vi "运维调试_采配水V1.vi"() -> ()   [LabVIEW 2016, in "PLC.lvlib"]
uses:
  PLC.lvlib
  <vilib>/Plasmionique/MB Master/MB_Master/MB_Master.lvclass
  <vilib>/Utility/miscctls.llb/LVPointTypeDef.ctl
  <vilib>/Plasmionique/MB Master/MB_Master_Serial/MB_Master_Serial.lvclass
  C:/Program Files (x86)/National Instruments/LabVIEW 2016/vi.lib/Plasmionique/MB Master/MB_Master/MB_Master.lvclass
  <vilib>/Instr/_visa.llb/VISA Configure Serial Port (Instr).vi
  <vilib>/NI/Modbus Library/API/Wrapper/Create TCP Slave.vi
  <vilib>/NI/Modbus Library/API/Slave/Modbus Slave.lvclass
  <vilib>/Plasmionique/MB Master/MB Master.lvlib
  <vilib>/NI/Modbus Library/API/Wrapper/API Main.lvlib
panel:
  out "Registers":u16[](array[numeric])
  out "R118":i16 caption="多参数沉淀时间"
  in  "下载模式":bool
  out "当前启动泵号":u16(ring) items=["1号水样泵", "2号水样泵"]
  out "R113":i16 caption="储水时间设定"
  out "X2":bool caption="X1"
  out "采配水版本号":string
  out "R23":i16 caption="清洗频次计数"
  out "R112":i16 caption="清洗频次设定"
  out "R22":i16
  in  "Y15":bool
  out "R111":i16 caption="排液时间"
  out "通讯故障":bool
  out "R21":i16
  in  "Y14":bool
  out "R20":i16
  in  "Y13":bool
  in  "潜水泵工作模式":u16(ring) items=["泵1单泵单管路", "泵2单泵单管路", "潜水泵双泵双管路", "自吸泵双泵双管路"]
  out "X10":bool caption="废液报警"
  out "X9":bool caption="自来水检测"
  out "X8":bool caption="泵2过载报警"
  out "X7":bool caption="泵1过载报警"
  out "X6":bool caption="断电检测"
  out "X5":bool caption="开门检测"
  out "X4":bool caption="烟雾检测"
  out "X3":bool caption="漏水检测"
  out "X1":bool
  out "X0":bool caption="采样池液位开关"
  out "R109":i16 caption="配水时间"
  out "集成报警信息":string
  out "R108":i16 caption="自来水报警"
  out "R107":i16 caption="采水池液位报警设置"
  out "R106":i16 caption="进样超时设置"
  out "R105":i16 caption="二级清洗时间"
  out "R104":i16 caption="一级清洗时间"
  out "R103":i16 caption="外部管路清洗时间"
  out "R102":i16 caption="静置沉淀时间"
  out "R101":i16 caption="内部管路润洗时间"
  out "R100":i16 caption="外部管路润洗时间"
  out "R2":i16
  out "R1":i16
  out "多列列表框":i32(listbox)
  out "R19":i16
  in  "Y7":bool
  out "R18":i16
  in  "Y6":bool
  out "R17":i16
  in  "Y5":bool
  out "R16":i16
  in  "Y4":bool
  out "R15":i16
  in  "Y3":bool
  out "R14":i16
  in  "Y2":bool
  out "R13":i16
  in  "Y1":bool
  out "R12":i16
  in  "Y0":bool
  in  "返回":bool
  in  "参数设置":bool
  in  "单步启动":bool
  in  "启动":bool
  in  "停止":bool
  # "S"
  # "S"
  # "次"
  # "次"
  # "S"
  # "S"
  # "S"
  # "S"
  # "S"
  # "S"
  # "S"
  # "S"
  # "S"
  # "S"
  # "S"
  # "单步计时："
  # "s"
  # "流程计时："
  # "s"
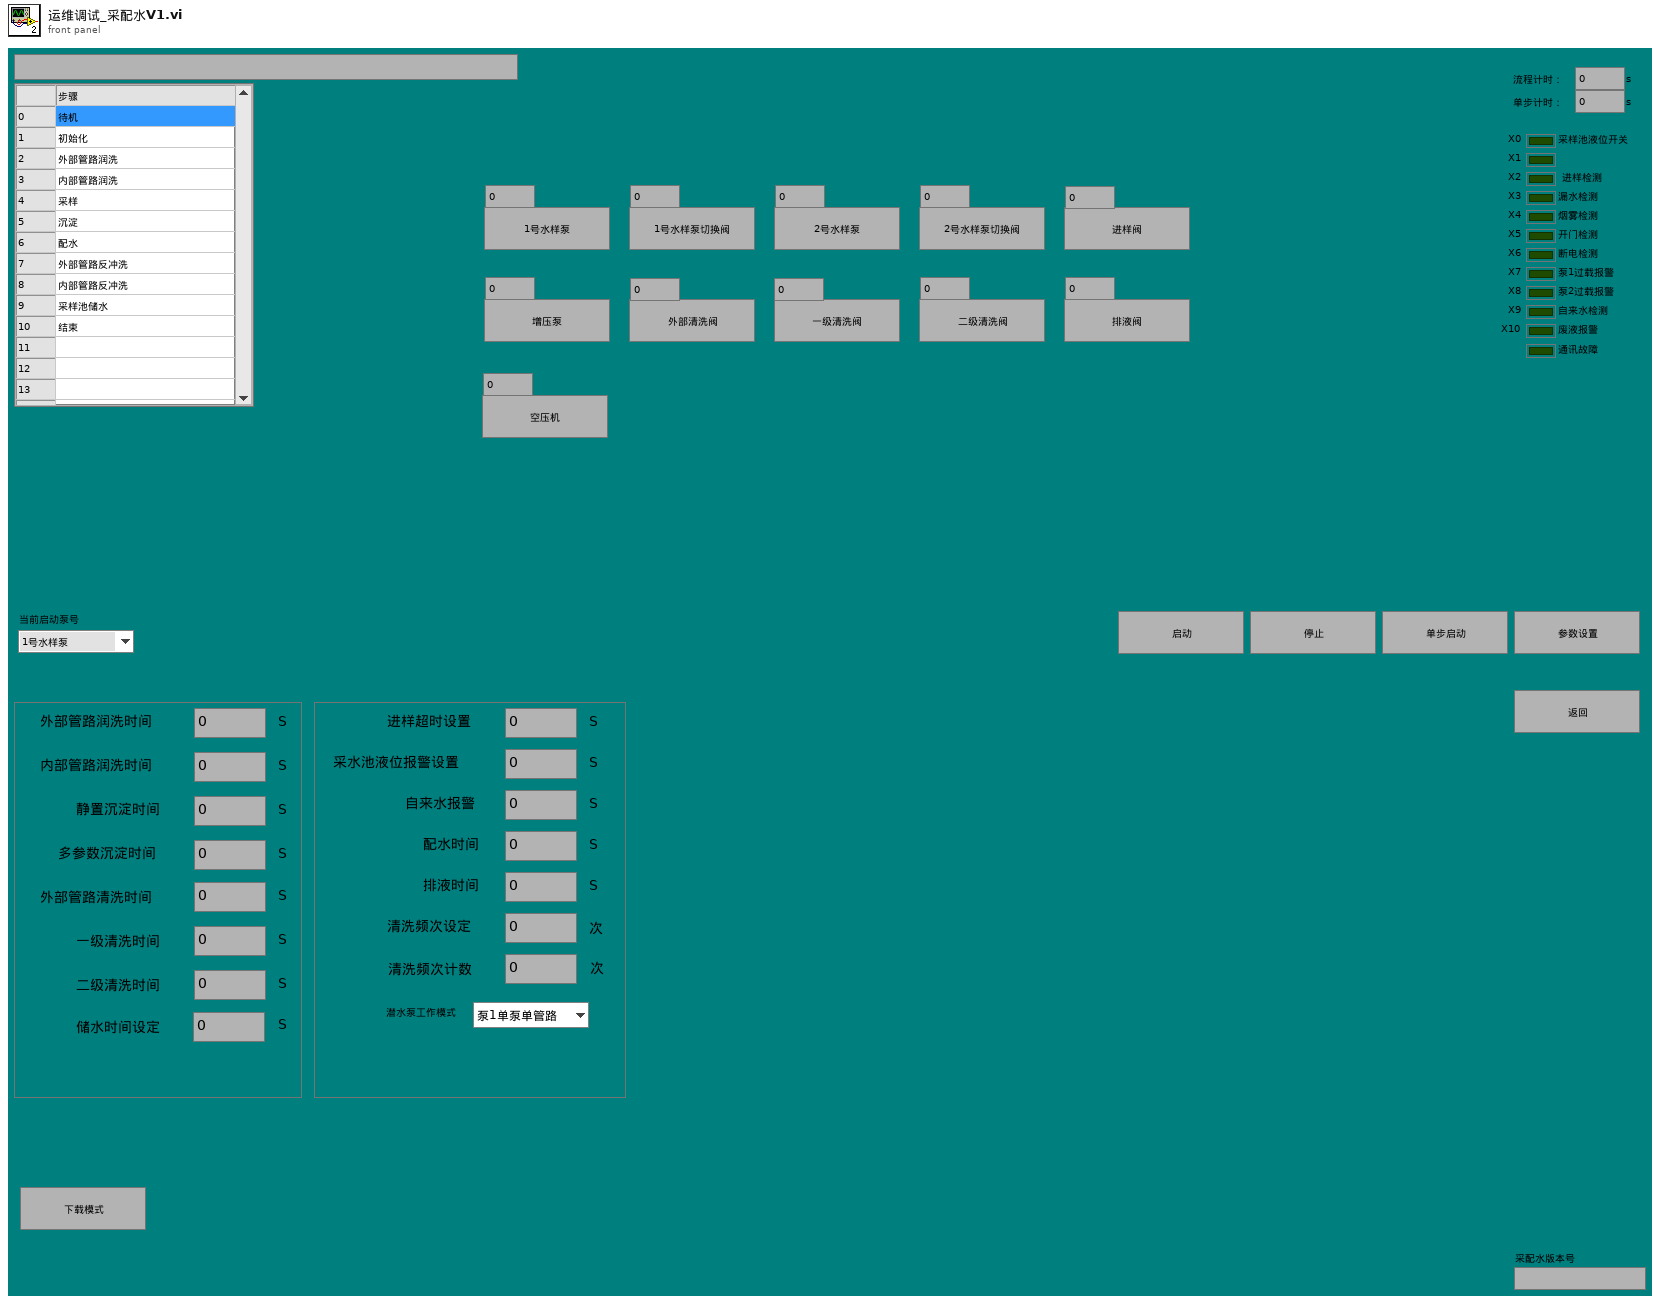
[diagram p1: front panel]
types:
  T1 = typedef "LVPointTypeDef.ctl" = cluster{"Horizontal":i16, "Vertical":i16}
  T2 = cluster{"命令":string, "数据":cluster{"starting address":u16, "holding register value":u16}}
  T3 = cluster{"时间标识":timestamp, "设备":string, "日志信息":string}
  T4 = cluster{"R0":i16, "R1":i16, "R2":i16, "R3":i16, "R4":i16, "R5":i16, "R6":i16, "R7":i16, "R8":i16, "R9":i16, "R10":i16, "R11":i16, "R12":i16, "R13":i16, "R14":i16, "R15":i16, "R16":i16, "R17":i16, "R18":i16, "R19":i16, "R20":i16, "R21":i16, "R22":i16, "R23":i16, "R24":i16, "R25":i16, "R26":i16, "R27":i16, "R28":i16, "R29":i16, "R30":i16, "R31":i16, "R32":i16, "R33":i16, "R34":i16}
  T5 = cluster{"seconds since 1Jan1904":timestamp, "table输入":string, string, "table输入":string}
  T6 = cluster{"时间标识":timestamp, "设备":string, "日志信息":string, "流程参数":string}
  T7 = cluster{"命令":string, cluster{"starting address":u16, "holding register value":u16}}
  T8 = cluster{"命令":string, "数据":cluster{"starting address":u16, "holding register values":u16[]}}
  T9 = cluster{"命令":string, "data":cluster{"starting address":u16, "coil values":bool[]}}
  T10 = cluster{"测试模式":enum16{"正常测试", "集成干预"}, "参数启用":cluster{"氨氮":bool, "总磷总氮":bool, "CODMn":bool, "CODcr":bool, "多参数":bool, "超标留样":bool}}
  T11 = enum32{"Bad", "Idle", "Run top level", "Running"}
  T12 = cluster{"baud rate (bps)":u32, "stop bits":u16, "parity":u16, "flow control":u16, "timeout":u32, "retries":i32}
  T13 = cluster{"starting address":u16, "holding register values":u16[]}
  T14 = cluster{"starting address":u16, "holding register value":u16}
  T15 = cluster{"starting address":u16, "coil values":bool[]}
  T16 = cluster{"Registers[0]":u16, "Registers[1]":u16, "Registers[2]":u16, "Registers[3]":u16, "Registers[4]":u16, "Registers[5]":u16, "Registers[6]":u16, "Registers[7]":u16, "Registers[8]":u16, "Registers[9]":u16, "Registers[10]":u16, "Registers[11]":u16, "Registers[12]":u16, "Registers[13]":u16, "Registers[14]":u16, "Registers[15]":u16, "Registers[16]":u16, "Registers[17]":u16, "Registers[18]":u16, "Registers[19]":u16, "Registers[20]":u16, "Registers[21]":u16, "Registers[22]":u16, "Registers[23]":u16, "Registers[24]":u16, "Registers[25]":u16, "Registers[26]":u16, "Registers[27]":u16, "Registers[28]":u16, "Registers[29]":u16, "Registers[30]":u16, "Registers[31]":u16, "Registers[32]":u16, "Registers[33]":u16, "Registers[34]":u16}
  T17 = cluster{"Registers[0]":u16, "Registers[1]":u16, "Registers[2]":u16, "Registers[3]":u16, "Registers[4]":u16, "Registers[5]":u16}
  T18 = cluster{"Registers[0]":u16, "Registers[1]":u16, "Registers[2]":u16, "Registers[3]":u16, "Registers[4]":u16, "Registers[5]":u16, "Registers[6]":u16, "Registers[7]":u16, "Registers[8]":u16, "Registers[9]":u16, "Registers[10]":u16, "Registers[11]":u16, "Registers[12]":u16, "Registers[13]":u16, "Registers[14]":u16, "Registers[15]":u16, "Registers[16]":u16, "Registers[17]":u16, "Registers[18]":u16, "Registers[19]":u16}
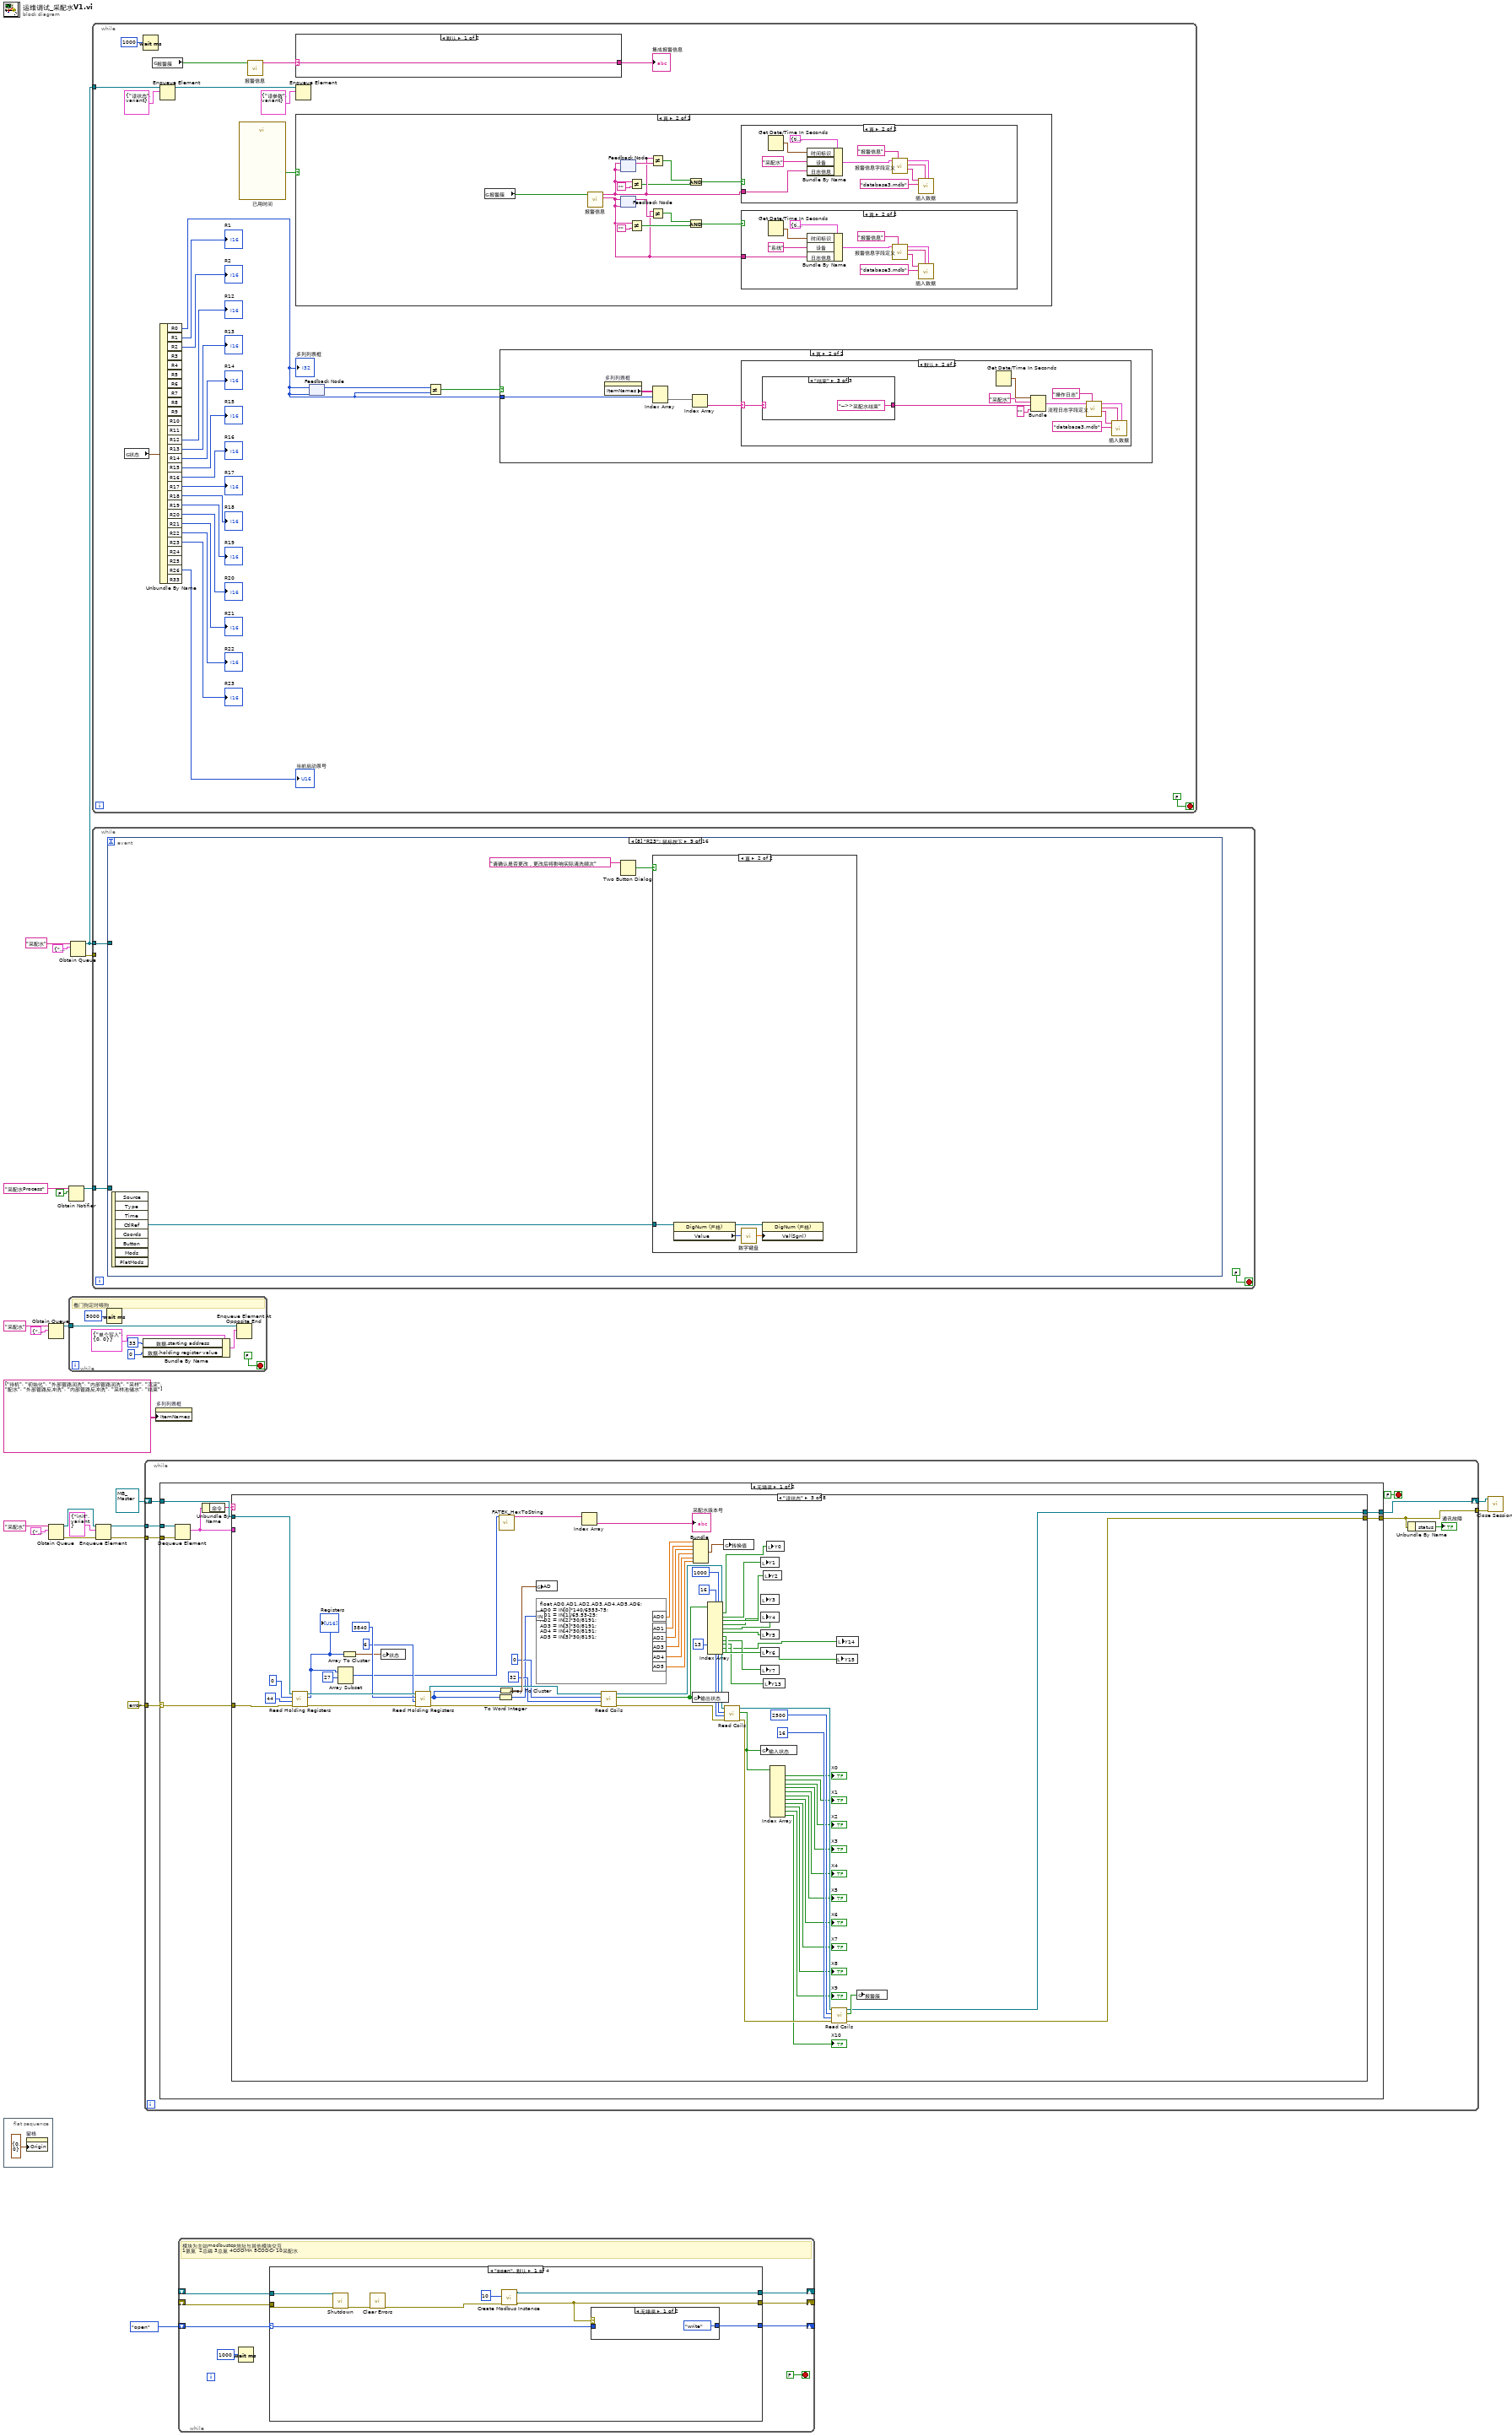
[diagram p0: block diagram]
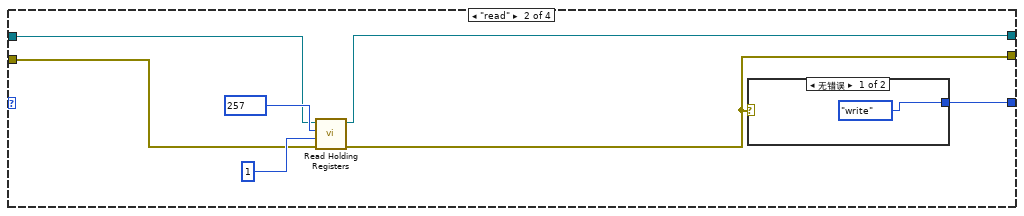
[diagram p3: hidden frame]
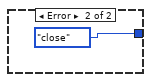
[diagram p4: hidden frame]
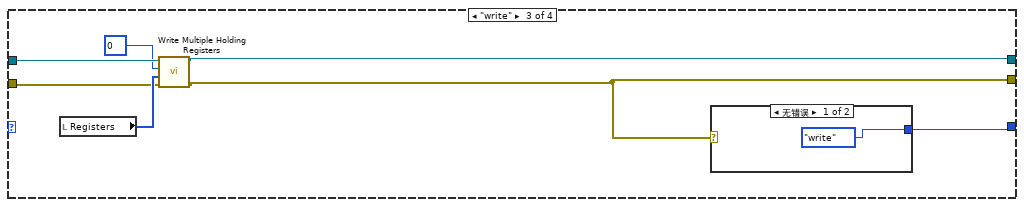
[diagram p5: hidden frame]
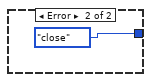
[diagram p6: hidden frame]
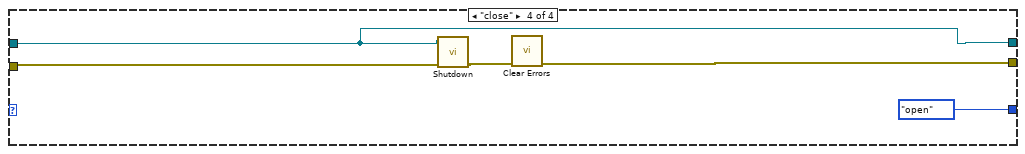
[diagram p7: hidden frame]
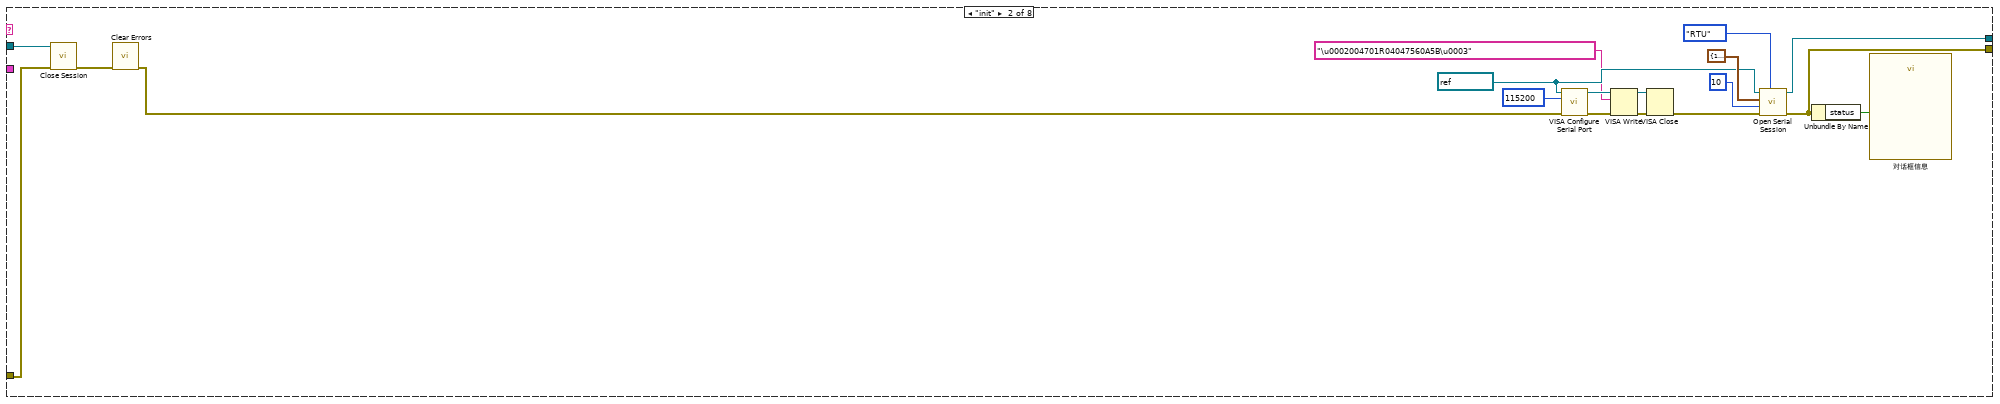
[diagram p9: hidden frame]
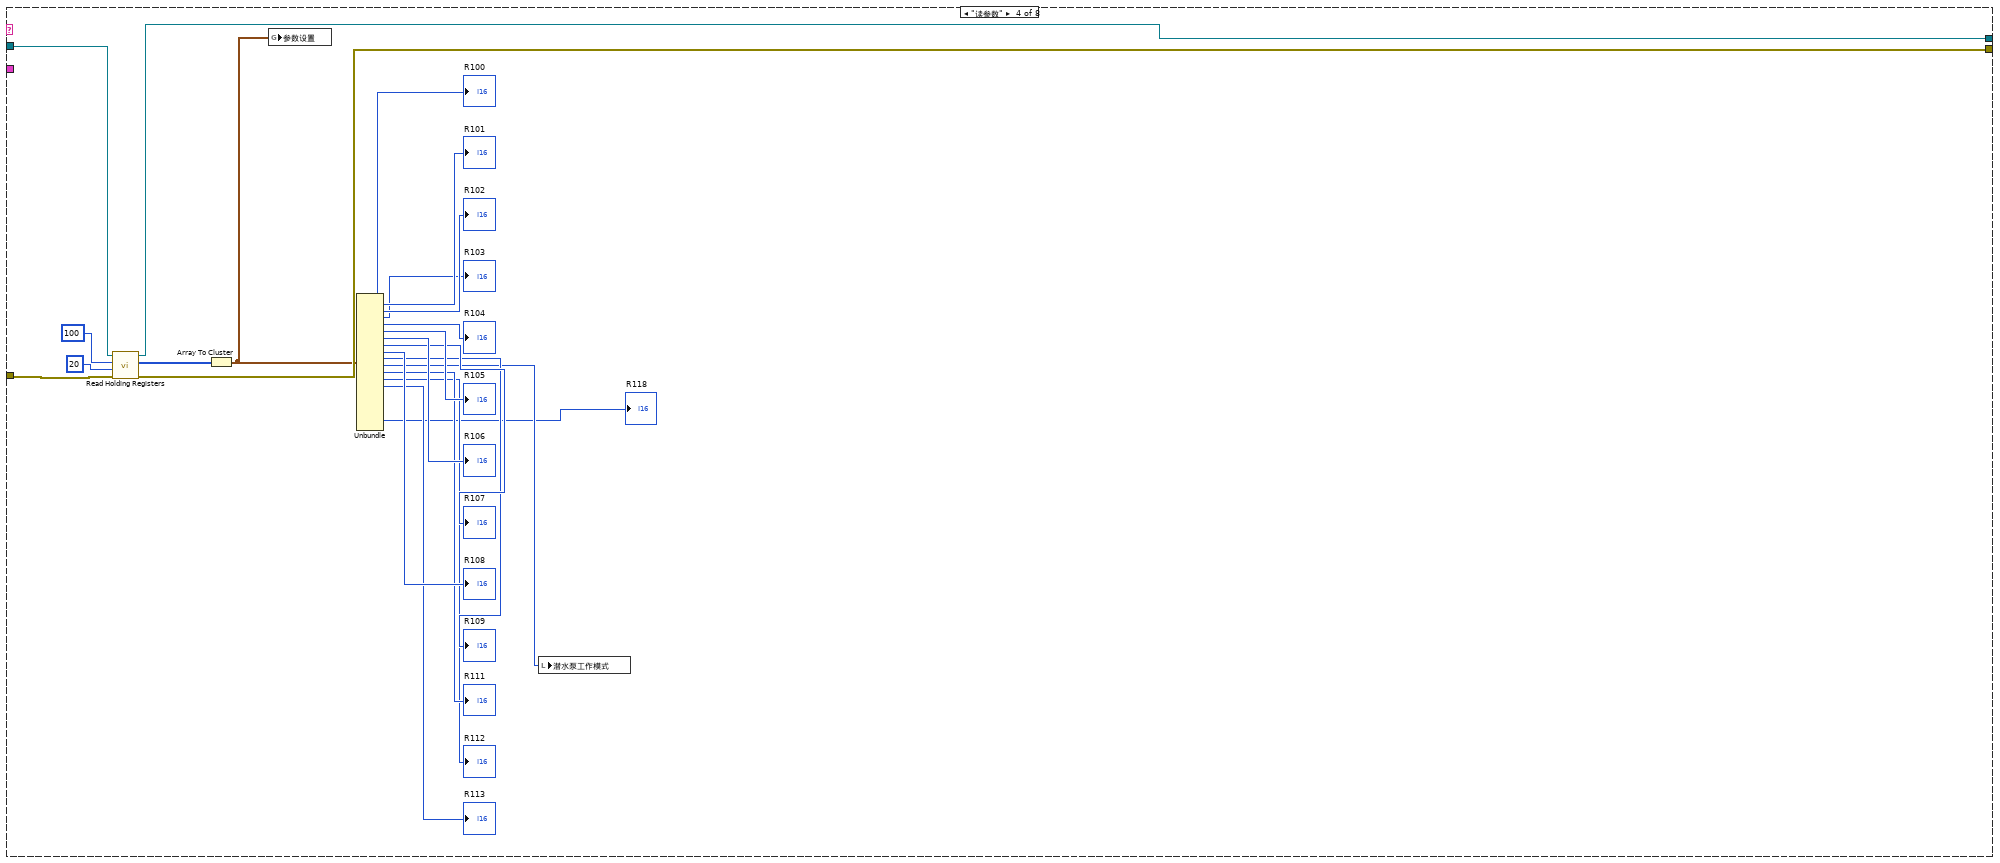
[diagram p10: hidden frame]
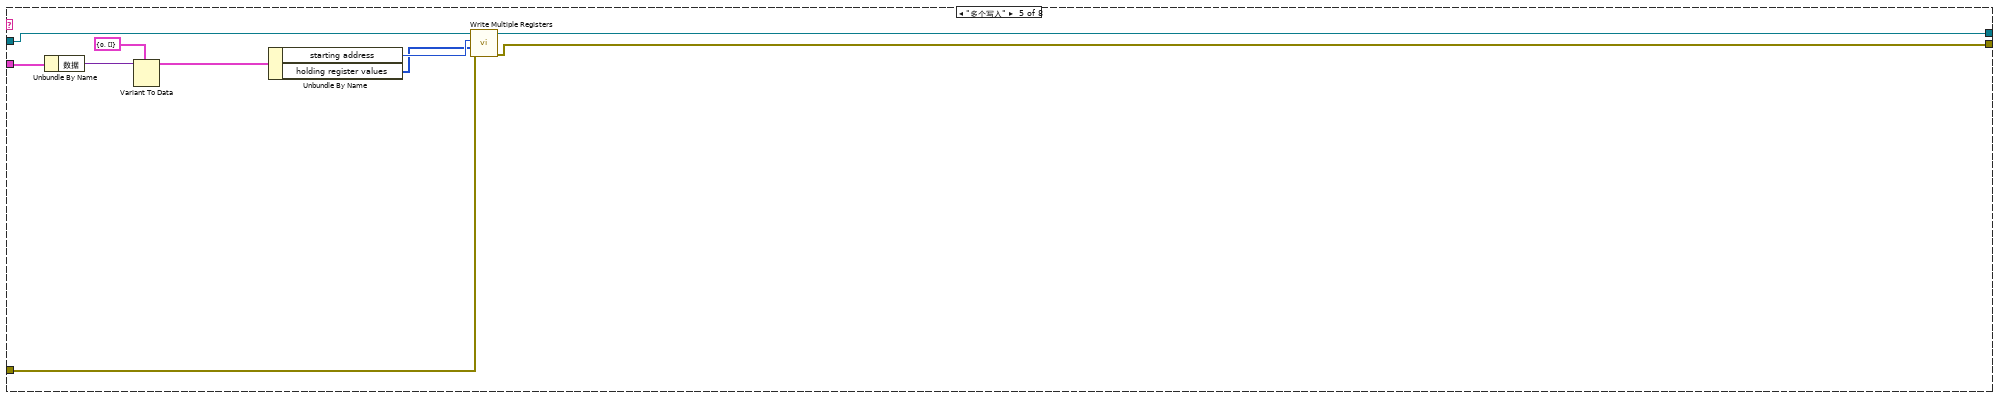
[diagram p11: hidden frame]
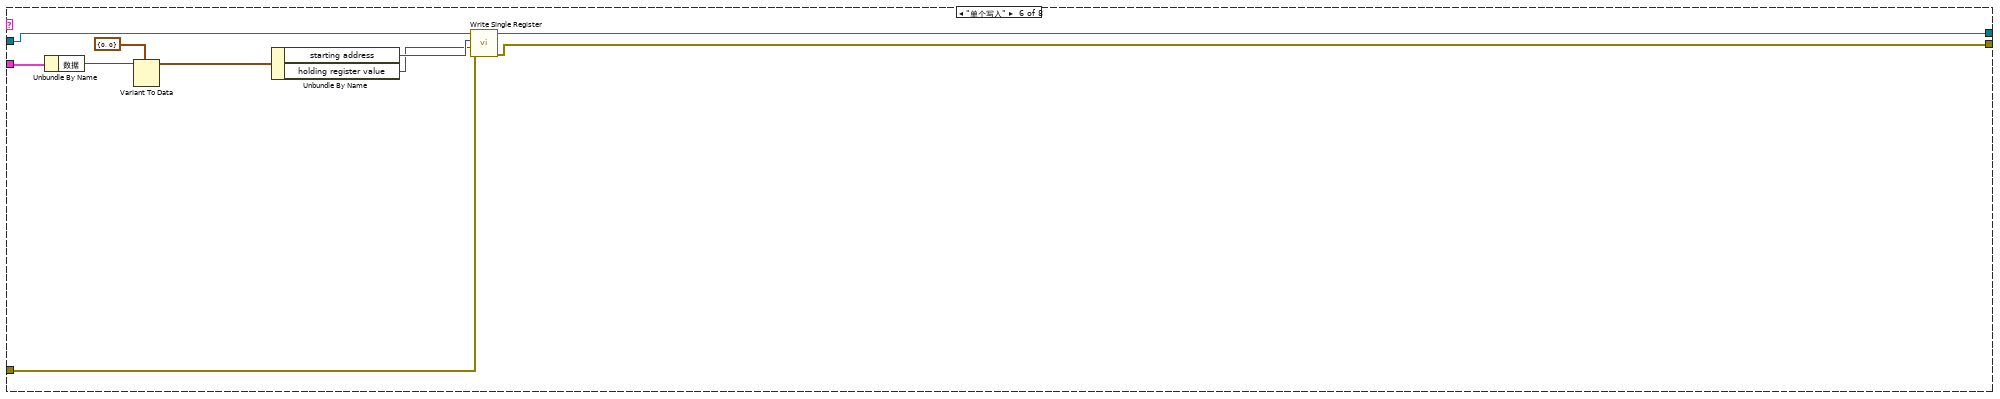
[diagram p12: hidden frame]
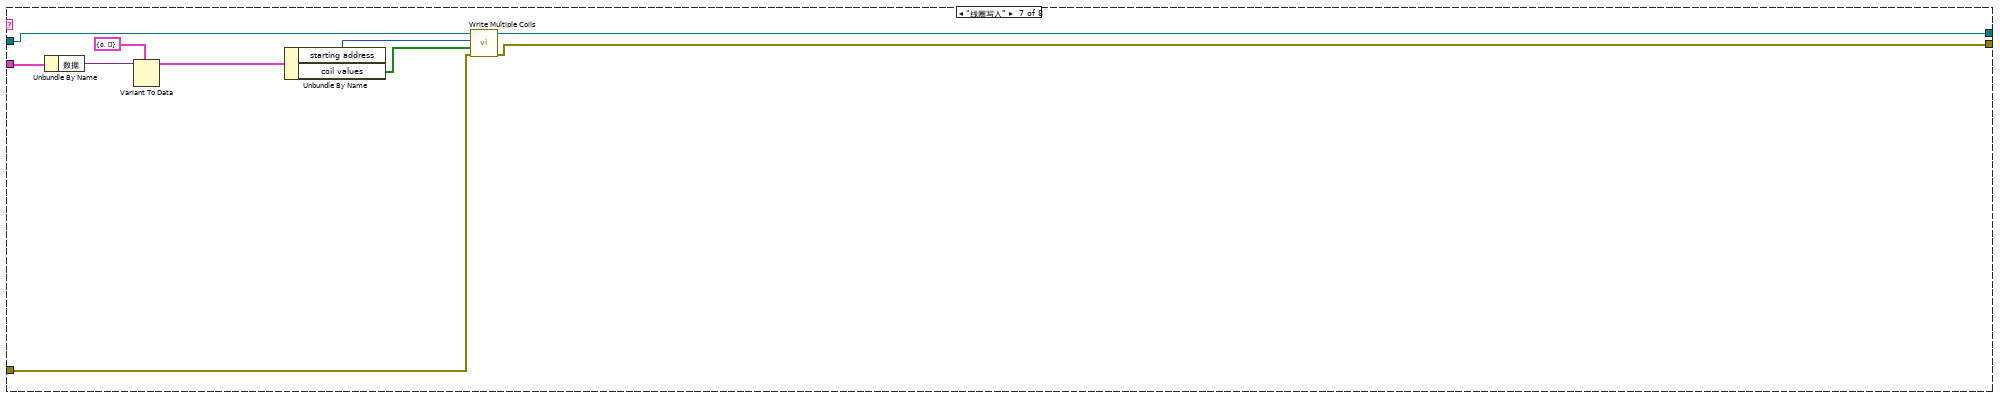
[diagram p13: hidden frame]
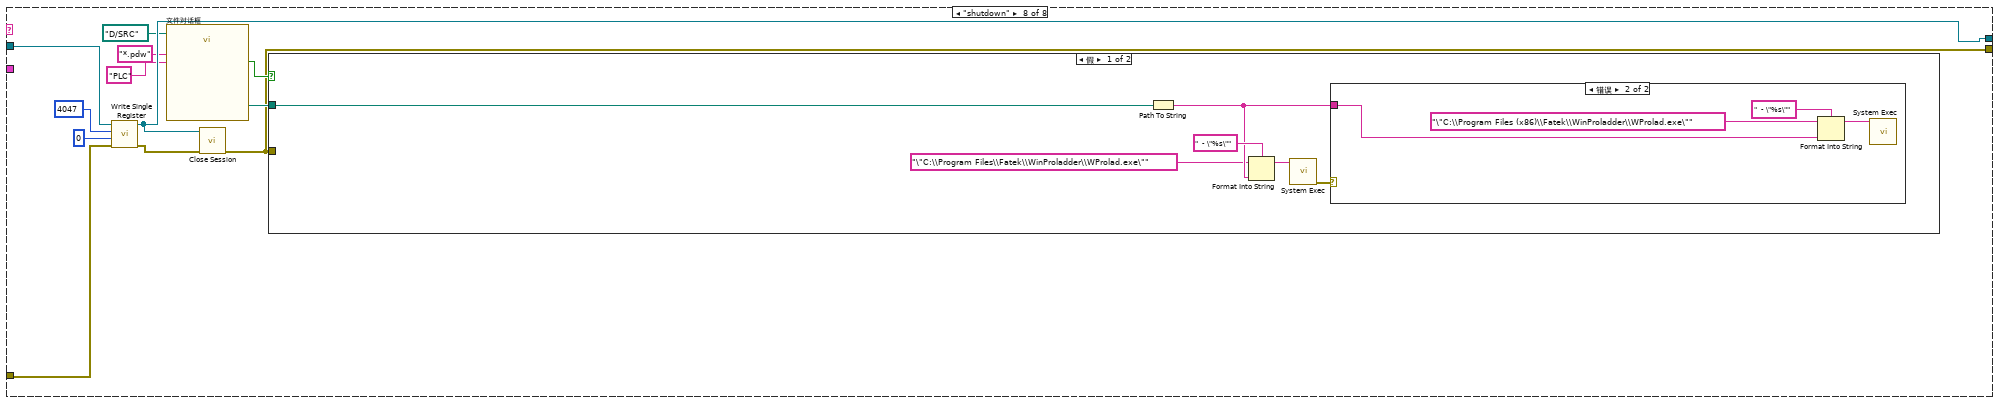
[diagram p14: hidden frame]
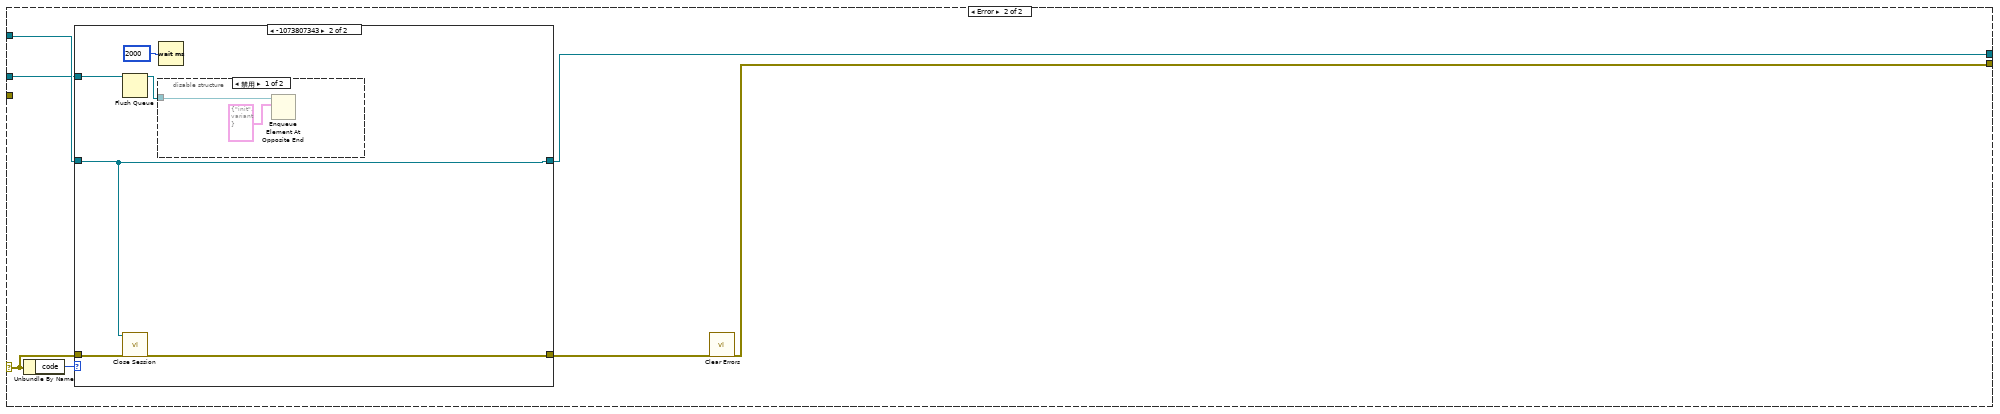
[diagram p17: hidden frame]
diagram:
  n1 = flat-sequence {
    frame #0 {
      n2 = property on="窗格" class="Pane"("Origin"=T1 {"Horizontal"=0, "Vertical"=0} ("原点")) -> ()  [unwired: 2 in, 2 out]
    }
  }
  n3 = Obtain Queue(name (unnamed)="采配水" ("名称（未命名）"), element data type=cluster{"命令":string, "数据":variant} {"命令"="", "数据"=variant}) -> (queue out=w2:refnum<queue>)  [unwired: 3 in, 2 out]
  n4 = Obtain Queue(name (unnamed)="采配水" ("名称（未命名）"), element data type=cluster{"命令":string, "数据":variant} {"命令"="", "数据"=variant}) -> (queue out=w13:refnum<queue>, error out=w12:errorcluster)  [unwired: 3 in, 1 out]
  n5 = Obtain Notifier(name (unnamed)="采配水Process" ("名称（未命名）"), notification data type=FALSE) -> (notifier out=w16:refnum<notifier>)  [unwired: 2 in, 2 out]
  n6 = while {
    tunnel: w2 -> [w27]
    stop <- FALSE stop-if-true
    # "看门狗定时喂狗"
    n7 = Wait (ms)(milliseconds to wait=u32 5000 ("等待时间（毫秒）")) -> ()  [unwired: 1 out]
    n8 = Bundle By Name(cluster=T2 {"命令"="单个写入", "数据"={"starting address"=0, "holding register value"=0}} ("元素"), "数据.starting address"=u16 33, "数据.holding register value"=u16 0) -> (w28:T2)
    n9 = Enqueue Element At Opposite End(queue=w27, element=w28) -> ()  [unwired: 2 in, 3 out]
  }
  n10 = Obtain Queue(name (unnamed)="采配水" ("名称（未命名）"), element data type=cluster{"命令":string, "数据":variant} {"命令"="", "数据"=variant}) -> (queue out=w20:refnum<queue>, error out=w21:errorcluster)  [unwired: 3 in, 1 out]
  n11 = while {
    tunnel: w20 -> [w59]
    stop <- FALSE stop-if-true
    n12 = global read "采配水全局变量.vi" "状态"() -> (w57:T4)
    n13 = Wait (ms)(milliseconds to wait=u32 1000 ("等待时间（毫秒）")) -> ()  [unwired: 1 out]
    n14 = global read "采配水全局变量.vi" "报警簇"() -> (w45:bool[])
    n15 = Enqueue Element(queue=w59, element=cluster{"命令":string, "数据":variant} {"命令"="读状态", "数据"=variant} ("元素")) -> (queue out=w40:refnum<queue>)  [unwired: 2 in, 2 out]
    n16 = Unbundle By Name(w57) -> ("R0"=w38:i16, "R1"=→"R1":i16, "R2"=→"R2":i16, "R12"=→"R12":i16, "R13"=→"R13":i16, "R14"=→"R14":i16, "R15"=→"R15":i16, "R16"=→"R16":i16, "R17"=→"R17":i16, "R18"=→"R18":i16, "R19"=→"R19":i16, "R20"=→"R20":i16, "R21"=→"R21":i16, "R22"=→"R22":i16, "R23"=→"R23":i16, "R26"=→"当前启动泵号":i16)  [unwired: 12 out]
    "多列列表框" <- w38
    n17 = call "已用时间"() -> ("Time has Elapsed"=w43:bool)  [unwired: 12 in, 7 out]
    n18 = call "报警信息.vi"("报警簇"=w45) -> ("采配水报警信息"=w37:string)  [unwired: 9 in, 1 out]
    n19 = case shown="默认" w37 {
      selector: w37 -> [w94 _]
      tunnel: [w94 w95] -> w44
      frame Default {
      }
      frame "" {
        n20 = global read "采配水全局变量.vi" "运行状态显示"() -> (w95:string)
      }
    }
    "集成报警信息" <- w44
    n21 = Enqueue Element(queue=w40, element=cluster{"命令":string, "数据":variant} {"命令"="读参数", "数据"=variant} ("元素")) -> ()  [unwired: 2 in, 3 out]
    n22 = case shown="真" w43 {
      frame False {
      }
      frame True {
        n23 = global read "采配水全局变量.vi" "报警簇"() -> (w73:bool[])
        n24 = call "报警信息.vi"("报警簇"=w73) -> ("系统报警信息"=w62:string, "采配水报警信息"=w69:string)  [unwired: 9 in]
        n25 = feedback #1(w69) -> (w72:string)
        n26 = feedback-in #1(w69) -> ()
        n27 = feedback #2(w62) -> (w63:string)
        n28 = feedback-in #2(w62) -> ()
        n29 = Not Equal?(x=w69, y="") -> (x != y?=w67:bool)
        n30 = Not Equal?(x=w62, y="") -> (x != y?=w66:bool)
        n31 = Not Equal?(x=w69, y=w72) -> (x != y?=w71:bool)
        n32 = Not Equal?(x=w62, y=w63) -> (x != y?=w64:bool)
        n33 = And(x=w71, y=w67) -> (x .and. y?=w70:bool)
        n34 = And(x=w64, y=w66) -> (x .and. y?=w61:bool)
        n35 = case shown="真" w70 {
          tunnel: w69 -> [_ w84]
          frame False {
          }
          frame True {
            n36 = Get Date/Time In Seconds() -> (seconds since 1Jan1904=w86:timestamp)
            n37 = Bundle By Name(cluster=T3 {"时间标识"=timestamp(0 s since 1904-01-01), "设备"="", "日志信息"=""} ("data in"), "时间标识"=w86, "设备"="采配水", "日志信息"=w84) -> (w87:T3)
            n38 = call "报警信息字段定义.vi"("table输入"="报警信息", "data in"=w87) -> ("table输出"=w91:string, "columns"=w92:string[], "data out"=w93:T3)  [unwired: 7 in]
            n39 = call "插入数据.vi"("data"=w93, "columns"=w92, "database"="database3.mdb", "table"=w91) -> ()  [unwired: 7 in, 1 out]
          }
        }
        n40 = case shown="真" w61 {
          tunnel: w62 -> [_ w74]
          frame False {
          }
          frame True {
            n41 = Get Date/Time In Seconds() -> (seconds since 1Jan1904=w76:timestamp)
            n42 = Bundle By Name(cluster=T3 {"时间标识"=timestamp(0 s since 1904-01-01), "设备"="", "日志信息"=""} ("data in"), "时间标识"=w76, "设备"="系统", "日志信息"=w74) -> (w77:T3)
            n43 = call "报警信息字段定义.vi"("table输入"="报警信息", "data in"=w77) -> ("table输出"=w81:string, "columns"=w82:string[], "data out"=w83:T3)  [unwired: 7 in]
            n44 = call "插入数据.vi"("data"=w83, "columns"=w82, "database"="database3.mdb", "table"=w81) -> ()  [unwired: 7 in, 1 out]
          }
        }
      }
    }
    n45 = feedback-in #3(w38) -> ()
    n46 = feedback #3(w38) -> (w39:i16)
    n47 = Not Equal?(x=w39, y=w38) -> (x != y?=w46:bool)
    n48 = case shown="真" w46 {
      tunnel: w38 -> [_ w98]
      frame False {
      }
      frame True {
        n49 = property on="多列列表框" class="MCListbox (严格)"() -> ("ItemNames"=w99:string[][])  [unwired: 2 in, 2 out]
        n50 = Index Array(array=w99, index (row)=w98) -> (element=w97:string[])  [unwired: 1 in]
        n51 = Index Array(array=w97) -> (element=w96:string)  [unwired: 1 in]
        n52 = case shown="默认" w96 {
          selector: w96 -> [_ w101]
          frame "待机" {
          }
          frame Default {
            n53 = case shown="\"结束\"" w101 {
              selector: w101 -> [w111 _ _]
              tunnel: [w111 "-->>采配水初始化" "-->>采配水结束"] -> w100
              frame Default {
              }
              frame "初始化" {
              }
              frame "结束" {
              }
            }
            n54 = Get Date/Time In Seconds() -> (seconds since 1Jan1904=w105:timestamp)
            n55 = Bundle("seconds since 1Jan1904"=w105, "table输入"="采配水", w100, "table输入"="") -> (w103:T5)  [unwired: 1 in]
            n56 = call "流程日志字段定义.vi"("table输入"="操作日志", "data in"=w103) -> ("table输出"=w108:string, "columns"=w109:string[], "data out"=w110:T6)  [unwired: 7 in]
            n57 = call "插入数据.vi"("data"=w110, "columns"=w109, "database"="database3.mdb", "table"=w108) -> ()  [unwired: 7 in, 1 out]
          }
        }
      }
    }
  }
  n58 = while {
    tunnel: w20 -> [w115]
    tunnel: w21 -> [_]
    tunnel: w16 -> [w114]
    stop <- FALSE stop-if-true
    n59 = event shown="[8] \"R23\": 鼠标按下" {
      selector: _ -> [_ _ _ _ _ _ _ _ _ _ _ _ _ _ _ _]
      dyn-events: _ -> [_ _ _ _ _ _ _ _ _ _ _ _ _ _ _ _]
      timeout: _ -> [_ _ _ _ _ _ _ _ _ _ _ _ _ _ _ _]
      tunnel: w115 -> [_ w119 w122 w144 w163 w166 w172 w183 _ _ _ _ w211 w213 w218 w223]
      tunnel: w114 -> [_ w118 w121 _ _ _ _ _ _ _ _ _ _ _ _ _]
      event Timeout {
        n60 = event-data() -> ()  [unwired: 1 in, 3 out]
      }
      event "停止": Value Change {
        n61 = event-data() -> ()  [unwired: 1 in, 6 out]
        n62 = Send Notification(notification=TRUE ("通知"), notifier=w118) -> ()  [unwired: 1 in, 2 out]
        n63 = Enqueue Element At Opposite End(queue=w119, element=T7 {"命令"="单个写入", {"starting address"=300, "holding register value"=2}} ("元素")) -> ()  [unwired: 2 in, 3 out]
      }
      event "启动": Value Change {
        n64 = event-data() -> ()  [unwired: 1 in, 6 out]
        n65 = disable-structure shown="禁用" {
          disable-tunnel: w122 -> [w140 _]
          frame Disabled {
            n66 = Enqueue Element At Opposite End(queue=w140, element=T7 {"命令"="单个写入", {"starting address"=300, "holding register value"=1}} ("元素")) -> ()  [unwired: 2 in, 3 out]
          }
          frame Enabled {
          }
        }
        n67 = flat-sequence {
          tunnel: w121 -> [w123]
          frame #0 {
            n68 = Cancel Notification(0:w123) -> ()  [unwired: 1 in, 3 out]
          }
          frame #1 {
            n69 = call "手动启动选择对话框.vi"() -> ("确定"=w125:bool, "参数"=w124:T10)  [unwired: 10 in]
            n70 = case shown="真" w125 {
              tunnel: w124 -> [_ w126]
              frame False {
              }
              frame True {
                n71 = vi-ref "PLC.lvlib:一体站流程自动启动.vi"() -> (w129:refnum<vi>)
                n72 = property class="VI"(reference=w129) -> ("Name"=w128:string, "Exec.State"=w127:T11)  [unwired: 1 in, 2 out]
                n73 = case shown="\"Idle\"" w127 {
                  tunnel: w128 -> [_ w137 _ _]
                  tunnel: w126 -> [_ w131 _ _]
                  frame "Bad", Default {
                  }
                  frame "Idle" {
                    n74 = Open VI Reference(type specifier VI Refnum (for type only)=refnum<vi> refnum, vi path=w137, options=128 ("选项")) -> (vi reference=w135:refnum<vi>, error out=w133:errorcluster)  [unwired: 3 in]
                    n75 = call-by-ref "开始异步调用"(reference=w135, error in=w133, "参数"=w131) -> (reference out=w134:refnum<vi>, error out=w132:errorcluster)  [unwired: 11 in]
                    n76 = Close Reference(reference=w134, error in (no error)=w132) -> ()  [unwired: 1 out]
                  }
                  frame "Run top level" {
                  }
                  frame "Running" {
                    n77 = One Button Dialog(message="流程已经运行,无须重复启动" ("消息")) -> ()  [unwired: 1 in, 1 out]
                  }
                }
              }
            }
          }
        }
      }
      event "单步启动": Value Change {
        n78 = event-data() -> ()  [unwired: 1 in, 6 out]
        n79 = call "单步启动对话框.vi"() -> ("单步启动步骤输出"=w141:u16)  [unwired: 11 in]
        n80 = Bundle By Name(cluster=T2 {"命令"="单个写入", "数据"={"starting address"=301, "holding register value"=0}} ("元素"), "数据.holding register value"=w141) -> (w142:T2)
        n81 = Enqueue Element At Opposite End(queue=w144, element=w142) -> ()  [unwired: 2 in, 3 out]
      }
      event "R100", "R101", "R102", "R103", "R104", "R105", "R106", "R107", "R108", "R109", "潜水泵工作模式", "R111", "R112", "R113": Value Change {
        n82 = event-data() -> ()  [unwired: 1 in, 6 out]
        n83 = local read "R100"() -> (w158:i16)
        n84 = local read "R101"() -> (w157:i16)
        n85 = local read "R102"() -> (w156:i16)
        n86 = local read "R103"() -> (w155:i16)
        n87 = local read "R104"() -> (w154:i16)
        n88 = local read "R105"() -> (w153:i16)
        n89 = local read "R106"() -> (w152:i16)
        n90 = local read "R107"() -> (w151:i16)
        n91 = local read "R108"() -> (w150:i16)
        n92 = local read "R109"() -> (w149:i16)
        n93 = local read "R111"() -> (w147:i16)
        n94 = local read "R112"() -> (w146:i16)
        n95 = local read "R113"() -> (w145:i16)
        n96 = Build Array(w158, w157, w156, w155, w154, w153, w152, w151, w150, w149, "潜水泵工作模式", w147, w146, w145) -> (w159:u16[])
        n97 = Bundle By Name(cluster=T8 {"命令"="多个写入", "数据"={"starting address"=0, "holding register values"=[]}} ("元素"), "数据.starting address"=u16 100, "数据.holding register values"=w159) -> (w160:T8)
        n98 = Enqueue Element At Opposite End(queue=w163, element=w160) -> ()  [unwired: 2 in, 3 out]
      }
      event "R118": Value Change {
        n99 = event-data() -> ()  [unwired: 1 in, 6 out]
        n100 = local read "R118"() -> (w164:i16)
        n101 = Build Array(w164) -> (w165:i16[])
        n102 = Bundle By Name(cluster=T8 {"命令"="多个写入", "数据"={"starting address"=0, "holding register values"=[]}} ("元素"), "数据.starting address"=u16 118, "数据.holding register values"=w165) -> (w167:T8)
        n103 = Enqueue Element At Opposite End(queue=w166, element=w167) -> ()  [unwired: 2 in, 3 out]
      }
      event "下载模式": Value Change {
        n104 = event-data() -> ("NewVal"=w171:bool)  [unwired: 1 in, 5 out]
        n105 = Flush Queue(queue=w172) -> (queue out=w170:refnum<queue>)  [unwired: 1 in, 2 out]
        n106 = case shown="真" w171 {
          tunnel: w170 -> [w173 w177]
          frame False {
            n107 = Enqueue Element At Opposite End(queue=w173, element=cluster{"命令":string, "数据":variant} {"命令"="init", "数据"=variant} ("元素")) -> ()  [unwired: 2 in, 3 out]
          }
          frame True {
            n108 = Two Button Dialog(message="请再次确认是否切换为下载模式，切换为下载模式将导致采配水工作异常，非专业人员请勿进行此操作！" ("消息")) -> (T button?=w175:bool)  [unwired: 2 in]
            n109 = case shown="真" w175 {
              tunnel: w177 -> [_ w180]
              frame False {
                n110 = local write "下载模式"(FALSE ("下载模式")) -> ()
              }
              frame True {
                n111 = Enqueue Element At Opposite End(queue=w180, element=cluster{"命令":string, "数据":variant} {"命令"="shutdown", "数据"=variant} ("元素")) -> ()  [unwired: 2 in, 3 out]
              }
            }
          }
        }
      }
      event "R23": Value Change {
        n112 = event-data() -> ()  [unwired: 1 in, 6 out]
        n113 = local read "R23"() -> (w182:i16)
        n114 = Build Array(w182) -> (w181:i16[])
        n115 = Bundle By Name(cluster=T8 {"命令"="多个写入", "数据"={"starting address"=0, "holding register values"=[]}} ("元素"), "数据.starting address"=u16 23, "数据.holding register values"=w181) -> (w184:T8)
        n116 = Enqueue Element At Opposite End(queue=w183, element=w184) -> ()  [unwired: 2 in, 3 out]
      }
      event "R23": Mouse Down {
        n117 = event-data() -> ("CtlRef"=w189:refnum<vi>)  [unwired: 1 in, 7 out]
        n118 = Two Button Dialog(message="请确认是否更改，更改后将影响实际清洗频次" ("消息")) -> (T button?=w188:bool)  [unwired: 2 in]
        n119 = case shown="真" w188 {
          tunnel: w189 -> [_ w190]
          frame False {
          }
          frame True {
            n120 = property class="DigNum (严格)"(reference=w190) -> (reference out=w192:refnum<vi>, "Value"=w193:i16)  [unwired: 1 in, 1 out]
            n121 = call "数字键盘.vi"("OldNumber"=w193) -> ("NewNumber"=w191:sgl)
            n122 = property class="DigNum (严格)"(reference=w192, "Val(Sgnl)"=w191) -> ()  [unwired: 1 in, 2 out]
          }
        }
      }
      event "R100", "R101", "R102", "R103", "R104", "R105", "R106", "R107", "R108", "R109", "R111", "R112", "R113", "R118": Mouse Down {
        n123 = event-data() -> ("CtlRef"=w197:refnum<vi>)  [unwired: 1 in, 7 out]
        n124 = property class="DigNum (严格)"(reference=w197) -> (reference out=w195:refnum<vi>, "Value"=w196:i16)  [unwired: 1 in, 1 out]
        n125 = call "数字键盘.vi"("OldNumber"=w196) -> ("NewNumber"=w194:sgl)
        n126 = property class="DigNum (严格)"(reference=w195, "Val(Sgnl)"=w194) -> ()  [unwired: 1 in, 2 out]
      }
      event "参数设置": Value Change {
        n127 = event-data() -> ()  [unwired: 1 in, 6 out]
        n128 = property on="窗格" class="Pane"("Origin"=T1 {"Horizontal"=0, "Vertical"=628} ("原点")) -> ()  [unwired: 2 in, 2 out]
      }
      event "返回": Value Change {
        n129 = event-data() -> ()  [unwired: 1 in, 6 out]
        n130 = property on="窗格" class="Pane"("Origin"=T1 {"Horizontal"=0, "Vertical"=0} ("原点")) -> ()  [unwired: 2 in, 2 out]
      }
      event "Y0", "Y1", "Y2", "Y3", "Y4", "Y5", "Y6", "Y7": Value Change {
        n131 = event-data() -> ()  [unwired: 1 in, 6 out]
        n132 = Build Array("Y0", "Y1", "Y2", "Y3", "Y4", "Y5", "Y6", "Y7") -> (w200:bool[])
        n133 = Bundle By Name(cluster=T9 {"命令"="线圈写入", "data"={"starting address"=2400, "coil values"=[]}} ("元素"), "data.coil values"=w200) -> (w201:T9)
        n134 = Enqueue Element(queue=w211, element=w201) -> ()  [unwired: 2 in, 3 out]
      }
      event "Y13": Value Change {
        n135 = event-data() -> ()  [unwired: 1 in, 6 out]
        n136 = Build Array("Y13") -> (w214:bool[])
        n137 = Bundle By Name(cluster=T9 {"命令"="线圈写入", "data"={"starting address"=2413, "coil values"=[]}} ("元素"), "data.coil values"=w214) -> (w215:T9)
        n138 = Enqueue Element(queue=w213, element=w215) -> ()  [unwired: 2 in, 3 out]
      }
      event "Y14": Value Change {
        n139 = event-data() -> ()  [unwired: 1 in, 6 out]
        n140 = Build Array("Y14") -> (w219:bool[])
        n141 = Bundle By Name(cluster=T9 {"命令"="线圈写入", "data"={"starting address"=2414, "coil values"=[]}} ("元素"), "data.coil values"=w219) -> (w220:T9)
        n142 = Enqueue Element(queue=w218, element=w220) -> ()  [unwired: 2 in, 3 out]
      }
      event "Y15": Value Change {
        n143 = event-data() -> ()  [unwired: 1 in, 6 out]
        n144 = Build Array("Y15") -> (w224:bool[])
        n145 = Bundle By Name(cluster=T9 {"命令"="线圈写入", "data"={"starting address"=2415, "coil values"=[]}} ("元素"), "data.coil values"=w224) -> (w225:T9)
        n146 = Enqueue Element(queue=w223, element=w225) -> ()  [unwired: 2 in, 3 out]
      }
    }
  }
  n147 = Enqueue Element(queue=w13, element=cluster{"命令":string, "数据":variant} {"命令"="init", "数据"=variant} ("元素"), error in (no error)=w12) -> (queue out=w8:refnum<queue>, error out=w10:errorcluster)  [unwired: 1 in, 1 out]
  n148 = while {
    tunnel: w8 -> [w231]
    tunnel: w10 -> [w230]
    shift-right: [w234] -> w5
    shift-left: refnum<class "MB_Master.lvclass"> refnum ("MB session in") -> [w233]
    tunnel: errorcluster {"status"=FALSE, "code"=0, "source"=""} ("error out") -> [w232]
    tunnel: [w229] -> w6
    stop <- FALSE stop-if-true
    n149 = case shown="无错误" w232 {
      selector: w232 -> [w239 w406]
      tunnel: [w242 w405] -> w234
      tunnel: w233 -> [w241 w407]
      tunnel: [w240 w403] -> w229
      tunnel: w231 -> [w237 w402]
      tunnel: w230 -> [w236 _]
      frame No Error {
        n150 = Dequeue Element(queue=w237, error in (no error)=w236) -> (element=w235:cluster{"命令":string, "数据":variant})  [unwired: 1 in, 3 out]
        n151 = Unbundle By Name(w235) -> ("命令"=w238:string)
        n152 = case shown="\"读状态\"" w238 {
          tunnel: [w244 w257 w277 w344 w356 w366 w376 w388] -> w242
          tunnel: w241 -> [w244 w259 w315 w349 w359 w369 w379 w391]
          tunnel: [w243 w258 w276 w343 w357 w367 w377 w382] -> w240
          tunnel: w239 -> [w243 w261 w318 w348 w358 w368 w378 w389]
          tunnel: w235 -> [_ _ _ _ w355 w365 w375 _]
          frame "idle", Default {
          }
          frame "init" {
            w249 = refnum<visa-resource-name> "COM3" ("VISA resource name")
            n153 = call-dynamic "Close Session.vi"("error in (no error)"=w261, "MB session in"=w259) -> ("error out"=w260:errorcluster)  [unwired: 9 in]
            n154 = call <vilib>:"Clear Errors.vi"("error in (no error)"=w260) -> ("error out"=w247:errorcluster)  [unwired: 5 in, 1 out]
            n155 = call-poly "VISA Configure Serial Port"("VISA resource name"=w249, "baud rate (9600)"=u32 115200, "error in (no error)"=w247) -> ("VISA resource name out"=w251:refnum<visa-resource-name>, "error out"=w253:errorcluster)  [unwired: 11 in]
            n156 = VISA Write(VISA resource name=w251, write buffer="\u0002004701R04047560A5B\u0003" ("写入缓冲区"), error in (no error)=w253) -> (VISA resource name out=w250:refnum<visa-resource-name>, error out=w252:errorcluster)  [unwired: 1 out]
            n157 = VISA Close(VISA resource name=w250, error in (no error)=w252) -> (error out=w246:errorcluster)
            n158 = call <vilib>:"Open Serial Session.vi"("Mode (RTU)"=enum16{"RTU", "ASCII"}."RTU", "Error in"=w246, "Slave ID"=u8 10, "Serial Config"=T12 {"baud rate (bps)"=115200, "stop bits"=10, "parity"=0, "flow control"=0, "timeout"=500, "retries"=1}, "VISA Resource"=w249) -> ("Error out"=w258:errorcluster, "MB_Serial session"=w257:refnum<class "MB_Master_Serial.lvclass">)  [unwired: 5 in]
            n159 = Unbundle By Name(w258) -> ("status"=w262:bool)
            n160 = call "对话框信息"("Enable"=w262) -> ()  [unwired: 9 in, 2 out]
          }
          frame "读状态" {
            n161 = call <vilib>:"Read Holding Registers.vi"("error in (no error)"=w318, "quantity"=u16 44 ("number of holding registers"), "starting address"=u16 0, "MB session in"=w315) -> ("error out"=w313:errorcluster, "Registers"=w274:u16[], "MB session out"=w314:refnum<class "MB_Master.lvclass">)  [unwired: 5 in]
            "Registers" <- w274
            n162 = Array Subset(array=w274, index=27 ("索引")) -> (w284:u16[])  [unwired: 1 in]
            n163 = Array To Cluster(array=w274) -> (cluster=w275:T16)
            n164 = global write "采配水全局变量.vi" "状态"(w275) -> ()
            n165 = call <vilib>:"Read Holding Registers.vi"("error in (no error)"=w313, "quantity"=u16 6 ("number of holding registers"), "starting address"=u16 3840, "MB session in"=w314) -> ("error out"=w309:errorcluster, "Registers"=w287:u16[], "MB session out"=w310:refnum<class "MB_Master.lvclass">)  [unwired: 5 in]
            n166 = To Word Integer(number=w287) -> (16bit integer=w286:i16[])
            n167 = call "FATEK_HexToString.vi"("数组"=w284) -> ("STRING"=w283:string[])  [unwired: 10 in]
            n168 = Array To Cluster(array=w287) -> (cluster=w326:T17)
            n169 = global write "采配水全局变量.vi" "AD"(w326) -> ()
            n170 = formula code="float AD0,AD1,AD2,AD3,AD4,AD5,AD6;\nAD0 = IN[0]*140/6553-75;\nAD1 = IN[1]/65.53-25;\nAD2 = IN[2]*30/8191;\nAD3 = IN[3]*30/8191;\nAD4 = IN[4]*30/8191;\nAD5 = IN[5]*30/8191;"("IN"=w286) -> ("AD0"=w324:dbl, "AD1"=w323:dbl, "AD2"=w322:dbl, "AD3"=w321:dbl, "AD4"=w320:dbl, "AD5"=w319:dbl)
            n171 = Index Array(array=w283) -> (element=→"采配水版本号":string)  [unwired: 1 in]
            n172 = call <vilib>:"Read Coils.vi"("error in (no error)"=w309, "quantity"=u16 32 ("number of coils"), "starting address"=u16 0, "MB session in"=w310) -> ("error out"=w305:errorcluster, "Coils"=w290:bool[], "MB session out"=w306:refnum<class "MB_Master.lvclass">)  [unwired: 5 in]
            n173 = global write "采配水全局变量.vi" "输出状态"(w290) -> ()
            n174 = Bundle(w324, w323, w322, w321, w320, w319) -> (w325:cluster{dbl, dbl, dbl, dbl, dbl, dbl})  [unwired: 1 in]
            n175 = Index Array(array=w290, index #9=13 ("索引")) -> (element #1=w273:bool, element #2=w281:bool, element #3=w272:bool, element #4=w271:bool, element #5=w270:bool, element #6=w269:bool, element #7=w268:bool, element #8=w267:bool, element #9=w265:bool, element #10=w264:bool, element #11=w263:bool)  [unwired: 10 in]
            n176 = global write "采配水全局变量.vi" "转换值"(w325) -> ()
            n177 = call <vilib>:"Read Coils.vi"("error in (no error)"=w305, "quantity"=u16 16 ("number of coils"), "starting address"=u16 1000, "MB session in"=w306) -> ("error out"=w301:errorcluster, "Coils"=w297:bool[], "MB session out"=w302:refnum<class "MB_Master.lvclass">)  [unwired: 5 in]
            n178 = local write "Y1"(w281) -> ()
            n179 = local write "Y3"(w271) -> ()
            n180 = local write "Y4"(w270) -> ()
            n181 = local write "Y5"(w269) -> ()
            n182 = local write "Y6"(w268) -> ()
            n183 = local write "Y7"(w267) -> ()
            n184 = global write "采配水全局变量.vi" "输入状态"(w297) -> ()
            n185 = local write "Y2"(w272) -> ()
            n186 = local write "Y13"(w265) -> ()
            n187 = local write "Y0"(w273) -> ()
            n188 = Index Array(array=w297) -> (element #1=→"X0":bool, element #2=→"X1":bool, element #3=→"X2":bool, element #4=→"X3":bool, element #5=→"X4":bool, element #6=→"X5":bool, element #7=→"X6":bool, element #8=→"X7":bool, element #9=→"X8":bool, element #10=→"X9":bool, element #11=→"X10":bool)  [unwired: 11 in]
            n189 = call <vilib>:"Read Coils.vi"("error in (no error)"=w301, "quantity"=u16 16 ("number of coils"), "starting address"=u16 2500, "MB session in"=w302) -> ("error out"=w276:errorcluster, "Coils"=w298:bool[], "MB session out"=w277:refnum<class "MB_Master.lvclass">)  [unwired: 5 in]
            n190 = local write "Y15"(w263) -> ()
            n191 = local write "Y14"(w264) -> ()
            n192 = global write "采配水全局变量.vi" "报警簇"(w298) -> ()
          }
          frame "读参数" {
            n193 = call <vilib>:"Read Holding Registers.vi"("error in (no error)"=w348, "quantity"=u16 20 ("number of holding registers"), "starting address"=u16 100, "MB session in"=w349) -> ("error out"=w343:errorcluster, "Registers"=w345:u16[], "MB session out"=w344:refnum<class "MB_Master.lvclass">)  [unwired: 5 in]
            n194 = Array To Cluster(array=w345) -> (cluster=w332:T18)
            n195 = global write "采配水全局变量.vi" "参数设置"(w332) -> ()
            n196 = Unbundle(w332) -> ("Registers[0]"=→"R100":u16, "Registers[1]"=→"R101":u16, "Registers[2]"=→"R102":u16, "Registers[3]"=→"R103":u16, "Registers[4]"=→"R104":u16, "Registers[5]"=→"R105":u16, "Registers[6]"=→"R106":u16, "Registers[7]"=→"R107":u16, "Registers[8]"=→"R108":u16, "Registers[9]"=→"R109":u16, "Registers[10]"=w331:u16, "Registers[11]"=→"R111":u16, "Registers[12]"=→"R112":u16, "Registers[13]"=→"R113":u16, "Registers[18]"=→"R118":u16)  [unwired: 5 out]
            n197 = local write "潜水泵工作模式"(w331) -> ()
          }
          frame "多个写入" {
            n198 = Unbundle By Name(w355) -> ("数据"=w354:variant)
            n199 = Variant To Data(type=T13 {"starting address"=0, "holding register values"=[]}, Variant=w354) -> (data=w352:T13)  [unwired: 1 in, 1 out]
            n200 = Unbundle By Name(w352) -> ("starting address"=w351:u16, "holding register values"=w350:u16[])
            n201 = call <vilib>:"Write Multiple Registers.vi"("error in (no error)"=w358, "values"=w350, "starting address"=w351, "MB session in"=w359) -> ("error out"=w357:errorcluster, "MB session out"=w356:refnum<class "MB_Master.lvclass">)  [unwired: 6 in]
          }
          frame "单个写入" {
            n202 = Unbundle By Name(w365) -> ("数据"=w364:variant)
            n203 = Variant To Data(type=T14 {"starting address"=0, "holding register value"=0}, Variant=w364) -> (data=w362:T14)  [unwired: 1 in, 1 out]
            n204 = Unbundle By Name(w362) -> ("starting address"=w361:u16, "holding register value"=w360:u16)
            n205 = call <vilib>:"Write Single Register.vi"("error in (no error)"=w368, "value"=w360, "address"=w361, "MB session in"=w369) -> ("error out"=w367:errorcluster, "MB session out"=w366:refnum<class "MB_Master.lvclass">)  [unwired: 6 in]
          }
          frame "线圈写入" {
            n206 = Unbundle By Name(w375) -> ("数据"=w374:variant)
            n207 = Variant To Data(type=T15 {"starting address"=0, "coil values"=[]}, Variant=w374) -> (data=w372:T15)  [unwired: 1 in, 1 out]
            n208 = Unbundle By Name(w372) -> ("starting address"=w371:u16, "coil values"=w370:bool[])
            n209 = call <vilib>:"Write Multiple Coils.vi"("error in (no error)"=w378, "values"=w370, "starting address"=w371, "MB session in"=w379) -> ("error out"=w377:errorcluster, "MB session out"=w376:refnum<class "MB_Master.lvclass">)  [unwired: 6 in]
          }
          frame "shutdown" {
            n210 = call <vilib>:"Write Single Register.vi"("error in (no error)"=w389, "value"=u16 0, "address"=u16 4047, "MB session in"=w391) -> ("error out"=w390:errorcluster, "MB session out"=w388:refnum<class "MB_Master.lvclass">)  [unwired: 6 in]
            n211 = call "文件对话框"("start path"=path "D:/SRC", "pattern (all files)"="*.pdw", "pattern label"="PLC") -> ("selected path"=w385:path, "cancelled"=w383:bool)  [unwired: 9 in, 2 out]
            n212 = call-dynamic "Close Session.vi"("error in (no error)"=w390, "MB session in"=w388) -> ("error out"=w382:errorcluster)  [unwired: 9 in]
            n213 = case shown="假" w383 {
              tunnel: w385 -> [w396 _]
              tunnel: w382 -> [_ _]
              frame False {
                n214 = Path To String(path=w396) -> (string=w393:string)
                n215 = Format Into String(format string="  - \"%s\"" ("格式字符串"), initial string="\"C:\\Program Files\\Fatek\\WinProladder\\WProlad.exe\"" ("command line"), w393) -> (resulting string=w394:string)  [unwired: 1 in, 1 out]
                n216 = call <vilib>:"System Exec.vi"("command line"=w394) -> ("error out"=w397:errorcluster)  [unwired: 7 in, 3 out]
                n217 = case shown="错误" w397 {
                  tunnel: w393 -> [_ w400]
                  frame No Error {
                  }
                  frame Error {
                    n218 = Format Into String(format string="  - \"%s\"" ("格式字符串"), initial string="\"C:\\Program Files (x86)\\Fatek\\WinProladder\\WProlad.exe\"" ("command line"), w400) -> (resulting string=w398:string)  [unwired: 1 in, 1 out]
                    n219 = call <vilib>:"System Exec.vi"("command line"=w398) -> ()  [unwired: 7 in, 4 out]
                  }
                }
              }
              frame True {
              }
            }
          }
        }
      }
      frame Error {
        n220 = Unbundle By Name(w406) -> ("code"=w408:i32)
        n221 = case shown="-1073807343" w408 {
          tunnel: w407 -> [w410 w414]
          tunnel: w406 -> [w409 w416]
          tunnel: [w409 w415] -> w404
          tunnel: [w410 w414] -> w405
          tunnel: w402 -> [_ w413]
          frame Default {
          }
          frame -1073807343 {
            n222 = Flush Queue(queue=w413) -> (queue out=w412:refnum<queue>)  [unwired: 1 in, 2 out]
            n223 = call-dynamic "Close Session.vi"("error in (no error)"=w416, "MB session in"=w414) -> ("error out"=w415:errorcluster)  [unwired: 9 in]
            n224 = disable-structure shown="禁用" {
              disable-tunnel: w412 -> [w417 _]
              frame Disabled {
                n225 = Enqueue Element At Opposite End(queue=w417, element=cluster{"命令":string, "数据":variant} {"命令"="init", "数据"=variant} ("元素")) -> ()  [unwired: 2 in, 3 out]
              }
              frame Enabled {
              }
            }
            n226 = Wait (ms)(milliseconds to wait=u32 2000 ("等待时间（毫秒）")) -> ()  [unwired: 1 out]
          }
        }
        n227 = call <vilib>:"Clear Errors.vi"("error in (no error)"=w404) -> ("error out"=w403:errorcluster)  [unwired: 5 in, 1 out]
      }
    }
    n228 = Unbundle By Name(w229) -> ("status"=→"通讯故障":bool)
  }
  n229 = property on="多列列表框" class="MCListbox (严格)"("ItemNames"=string[][] [["待机"], ["初始化"], ["外部管路润洗"], ["内部管路润洗"], ["采样"], ["沉淀"], ["配水"], ["外部管路反冲洗"], ["内部管路反冲洗"], ["采样池储水"], ["结束"]] ("项名")) -> ()  [unwired: 2 in, 2 out]
  n230 = while {
    shift-right: [w424] -> _
    shift-left: _ -> [w426]
    shift-right: [w423] -> _
    shift-left: _ -> [w425]
    shift-right: [w420] -> _
    shift-left: enum16{"open", "read", "write", "close"}."open" -> [w421]
    stop <- FALSE stop-if-true
    # "模块为主站modbustcp地址与其他模块交互\n1氨氮  2总磷 3总氮 4CODMn 5CODCr 10采配水"
    n231 = Wait (ms)(milliseconds to wait=u32 1000 ("等待时间（毫秒）")) -> ()  [unwired: 1 out]
    n232 = case shown="\"open\", 默认" w421 {
      selector: w421 -> [w435 _ _ _]
      tunnel: w426 -> [w429 w441 w452 w458]
      tunnel: w425 -> [w428 w440 w449 w457]
      tunnel: [w432 w438 w448 w458] -> w424
      tunnel: [w431 w439 w447 w460] -> w423
      tunnel: [w434 w444 w453 enum16{"open", "read", "write", "close"}."open"] -> w420
      frame "open", Default {
        n233 = call-dynamic "Shutdown.vi"("error in"=w428, "Modbus slave in"=w429) -> ("error out"=w427:errorcluster)  [unwired: 9 in]
        n234 = call <vilib>:"Clear Errors.vi"("error in (no error)"=w427) -> ("error out"=w430:errorcluster)  [unwired: 5 in, 1 out]
        n235 = call-poly <vilib>:"Create Modbus Instance.vi"("error in"=w430, "port (502)"=u16 10) -> ("error out"=w431:errorcluster, "TCP slave instance"=w432:refnum<class "Modbus Slave.lvclass">)  [unwired: 8 in]
        n236 = case shown="无错误" w431 {
          tunnel: w435 -> [_ w437]
          tunnel: [enum16{"open", "read", "write", "close"}."write" w437] -> w434
          frame No Error {
          }
          frame Error {
          }
        }
      }
      frame "read" {
        n237 = call-dynamic <vilib>:"Read Holding Registers.vi"("error in"=w440, "number of inputs"=u16 1, "starting address"=u16 257, "Modbus slave in"=w441) -> ("error out"=w439:errorcluster, "Modbus slave out"=w438:refnum<class "Modbus Slave.lvclass">)  [unwired: 5 in, 1 out]
        n238 = case shown="无错误" w439 {
          tunnel: [enum16{"open", "read", "write", "close"}."write" enum16{"open", "read", "write", "close"}."close"] -> w444
          frame No Error {
          }
          frame Error {
          }
        }
      }
      frame "write" {
        n239 = local read "Registers"() -> (w450:u16[])
        n240 = call-dynamic "Write Multiple Holding Registers.vi"("error in"=w449, "registers to write"=w450, "starting address"=u16 0, "Modbus slave in"=w452) -> ("error out"=w447:errorcluster, "Modbus slave out"=w448:refnum<class "Modbus Slave.lvclass">)  [unwired: 6 in]
        n241 = case shown="无错误" w447 {
          tunnel: [enum16{"open", "read", "write", "close"}."write" enum16{"open", "read", "write", "close"}."close"] -> w453
          frame No Error {
          }
          frame Error {
          }
        }
      }
      frame "close" {
        n242 = call-dynamic "Shutdown.vi"("error in"=w457, "Modbus slave in"=w458) -> ("error out"=w456:errorcluster)  [unwired: 9 in]
        n243 = call <vilib>:"Clear Errors.vi"("error in (no error)"=w456) -> ("error out"=w460:errorcluster)  [unwired: 5 in, 1 out]
      }
    }
  }
  n244 = call-dynamic "Close Session.vi"("error in (no error)"=w6, "MB session in"=w5) -> ()  [unwired: 9 in, 1 out]
